vi "findleftmostbitI16.vi"(11 "number":i16 format="%b") -> (3 "Numeric":i16)   [LabVIEW 2018]
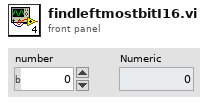
[diagram p1: front panel]
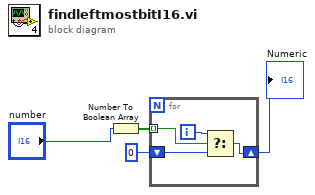
[diagram p0: block diagram]
diagram:
  n1 = Number To Boolean Array(number="number") -> (Boolean array=w2:bool[])
  n2 = for {
    tunnel: w2 -> [w8] mode=indexing
    shift-right: [w5] -> w3
    shift-left: 0 -> [w6]
    i -> [w7]
    n3 = Select(t=w7, s=w8, f=w6) -> (s? t:f=w5:i32)
  }
  "Numeric" <- w3
